vi "Read Configuration File.vi"(8 "error in (no error)":errorcluster, 11 "Instrument.Oxford1820 in":refnum<class "Instrument.Oxford1820.lvclass">) -> (0 "error out":errorcluster, 3 "Instrument.Oxford1820 out":refnum<class "Instrument.Oxford1820.lvclass">)   [LabVIEW 2019, in "Instrument.Oxford1820.lvclass"]
uses:
  Instrument.Oxford1820.lvclass
  C:/Program Files/National Instruments/LabVIEW 2019/user.lib/LevyLab/Instrument Framework/Instrument/Instrument.lvclass
  <userlib>/LevyLab/Instrument Framework/Instrument/Instrument.lvclass/Instrument.ctl
  <userlib>/LevyLab/Configuration/Configuration.lvclass/Configuration.ctl
  Instrument.Oxford1820.lvclass/Instrument.Oxford1820.ctl
  <userlib>/LevyLab/Configuration/Write Section.vi
  <userlib>/LevyLab/Instrument Framework/Instrument/Instrument.lvclass
  C:/Program Files/National Instruments/LabVIEW 2019/vi.lib/JKI/JKI SMO/SMO/SMO.lvclass
  <vilib>/JKI/JKI SMO/SMO/Protected/ThisLevelClassName.vi
  <userlib>/LevyLab/Instrument Framework/Instrument Types/Cryostat/Instrument.Cryostat.lvclass
  <userlib>/LevyLab/Configuration/Configuration.lvclass
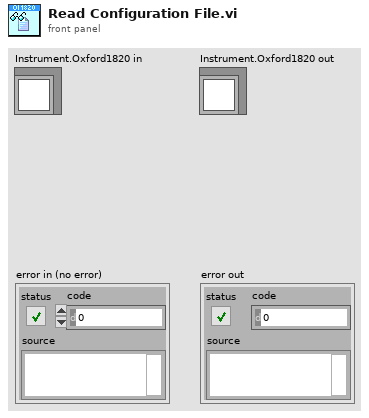
[diagram p1: front panel]
types:
  T1 = cluster{"IPS Address":string, "ITC Address":string}
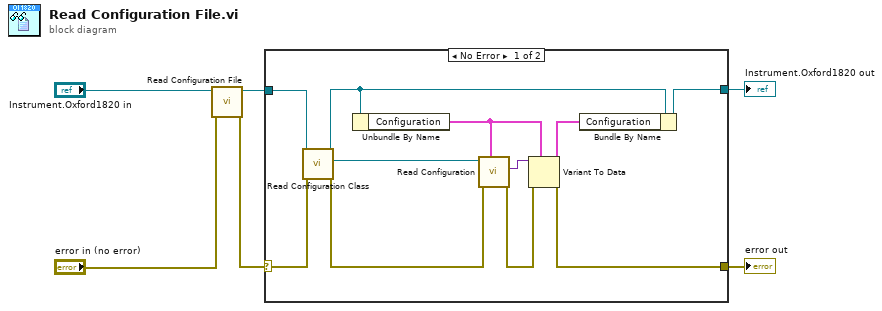
[diagram p0: block diagram]
diagram:
  n1 = call-parent "Read Configuration File.vi"("error in (no error)"="error in (no error)", "Instrument in"="Instrument.Oxford1820 in") -> ("error out"=w3:errorcluster, "Instrument out"=w4:refnum<class "Instrument.Oxford1820.lvclass">)  [unwired: 8 in]
  n2 = case shown="No Error" w3 {
    selector: w3 -> [w14 w19]
    tunnel: [w13 w19] -> w2
    tunnel: [w17 w18] -> w5
    tunnel: w4 -> [w16 w18]
    frame No Error {
      n3 = call <userlib>:"Read Configuration Class.vi"("error in (no error)"=w14, "Instrument in"=w16) -> ("error out"=w11:errorcluster, "Configuration"=w10:refnum<class "Configuration.lvclass">, "Instrument out"=w15:refnum<class "Instrument.Oxford1820.lvclass">)  [unwired: 7 in]
      n4 = Unbundle By Name(w15) -> ("Configuration"=w12:T1)
      n5 = call <userlib>:"Read Configuration.vi"("INI Fomatted Cluster Type"=w12, "error in (no error)"=w11, "Configuration in"=w10) -> ("error out"=w8:errorcluster, "Configuration"=w9:variant)  [unwired: 6 in, 1 out]
      n6 = Variant To Data(error in=w8, type=w12, Variant=w9) -> (data=w7:T1, error out=w13:errorcluster)
      n7 = Bundle By Name(cluster=w15, "Configuration"=w7) -> (w17:refnum<class "Instrument.Oxford1820.lvclass">)
    }
    frame Error {
    }
  }
  "Instrument.Oxford1820 out" <- w5
  "error out" <- w2
